vi "Mark Sensor Plots.vi"(0 "Segment Select Ref":refnum<vi>, 1 "Segement Start":dbl, 2 "End":dbl, 3 "Start":dbl) -> ()   [LabVIEW 2020]
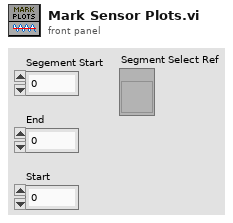
[diagram p1: front panel]
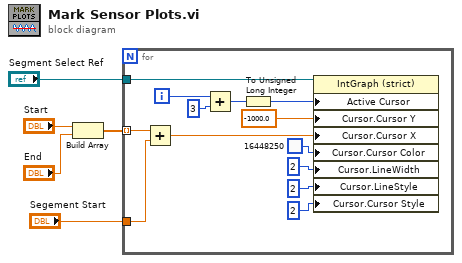
[diagram p0: block diagram]
diagram:
  n1 = Build Array("Start", "End") -> (w4:dbl[])
  n2 = for {
    tunnel: w4 -> [w11] mode=indexing
    tunnel: "Segement Start" -> [w10]
    tunnel: "Segment Select Ref" -> [w18]
    i -> [w8]
    n3 = Add(x=w11, y=w10) -> (x+y=w9:dbl)
    n4 = Add(x=w8, y=3) -> (x+y=w7:i32)
    n5 = To Unsigned Long Integer(number=w7) -> (unsigned 32bit integer=w13:u32)
    n6 = property class="IntGraph (strict)"(reference=w18, "Active Cursor"=w13, "Cursor.Cursor Y"=-1000.0 ("Cursor.Cursor Position:Cursor Y"), "Cursor.Cursor X"=w9, "Cursor.Cursor Color"=u32 16448250, "Cursor.LineWidth"=u8 2 ("Cursor.Line Width"), "Cursor.LineStyle"=u8 2 ("Cursor.Line Style"), "Cursor.Cursor Style"=u8 2) -> ()  [unwired: 1 in, 2 out]
  }
